vi "InjA-FPGA.vi"() -> ()   [LabVIEW 2016]
uses:
  Common-Control/Aperture Readback.ctl
  Common-Control/Glassman Readback.ctl
  Common-Control/Glassman Control.ctl
  <vilib>/LabVIEW Targets/FPGA/cRIO/shared/nicrio_ModuleControls/nicrio_cRIO-9871_BaudRateEnum.ctl
  <vilib>/LabVIEW Targets/FPGA/cRIO/shared/nicrio_ModuleControls/nicrio_cRIO-9871_DataBitsEnum.ctl
  <vilib>/LabVIEW Targets/FPGA/cRIO/shared/nicrio_ModuleControls/nicrio_cRIO-9871_ParityEnum.ctl
  <vilib>/LabVIEW Targets/FPGA/cRIO/shared/nicrio_ModuleControls/nicrio_cRIO-9871_StopBitsEnum.ctl
  <vilib>/Platform/TimedLoop/XDataNode/timing_clust.ctl
  <vilib>/Platform/TimedLoop/XDataNode/nitl_modes.ctl
  <vilib>/Platform/TimedLoop/XDataNode/wakeup.ctl
  <vilib>/rvi/FXPMathLib/basic elements/FxpIntAccumulator/subVIs/nifxpmath_IntAccumulator_SimConfig.ctl
  <vilib>/rvi/Emulation/niFpgaGetClockAttributes.vi
  <vilib>/rvi/Emulation/niFpgaSctlEmulationGetInTimedLoop.vi
  <vilib>/rvi/Emulation/niFpgaEmulationReportErrorSimple.vi
  <vilib>/rvi/eio/common/nirviEmuTemplateMethod_errors.vi
  <vilib>/rvi/Emulation/niFpgaCriticalErrorInLSC.vi
  <vilib>/rvi/Analysis/common/codeGenErrors/XNode/niFpgaXNodeCodeGenErrorHandle.vi
  <vilib>/rvi/FXPMathLib/basic elements/FxpIntAccumulator/simVIs/DllFxpIntAccumulator_sub.vi
  <vilib>/rvi/eio/common/nirviEmuTemplatePropertySet_errors.vi
  <vilib>/eio/EIONode/EIONode.xnode
  <vilib>/rvi/Analysis/measure/dc-rms/XNode/niFpgaDC-RMS.xnode
  <vilib>/Platform/TimedLoop/XDataNode/XDataNode.xnode
  <vilib>/rvi/FXPMathLib/basic elements/FxpIntAccumulator/XNode/nifxpmath_IntAccumulator.xnode
  <vilib>/rvi/FXPMathLib/FxpMul/XNode/nifxpmath_Multiplier.xnode
  <vilib>/eio/EIOPropertyNode/EIOPropertyNode.xnode
  <vilib>/Platform/TimedLoop/XDataNode/XDNodeRunTimeDep.lvlib
  <vilib>/rvi/FXPMathLib/sim/FxpSim.dll
  <vilib>/rvi/eio/common/nirviEmuTemplatePropertyGet_errors.vi
  <vilib>/rvi/eio/common/nirviEmuTemplatePropertyGet_noerrors.vi
  <vilib>/rvi/eio/common/nirviEmuTemplatePropertySet_noerrors.vi
panel:
  out "Turbo Rotation Status":bool
  out "Turbo Error Status":bool
  out "Turbo Rotation Speed":fxp<+/-,26,5>
  out "Turbo monitor loop error":errorcluster
  out "HV control loop error":errorcluster
  in  "Einzel 2 V set":T1
  in  "Y Steerer V set":T1
  in  "X Steerer V set":T1
  in  "Einzel 1 V set":T1
  out "HV readback loop error":errorcluster
  out "Y Steerer Monitor":T2
  out "X Steerer Monitor":T2
  out "Einzel 2 Monitor":T2
  out "Einzel 1 Monitor":T2
  out "Pre-Acc Aperture Position":T3
  in  "RT error":bool
  out "Vac readback loop error":errorcluster
  out "Ion gauge 1":u8[](array[numeric])
  out "Convectron 1":u8[](array[numeric])
  out "Ion gauge 2":u8[](array[numeric])
  out "Convectron 2":u8[](array[numeric])
  out "Vacuum Gauge interlock":bool
  out "Vac Interlock loop error":errorcluster
  out "Actuator Sensor loop error":errorcluster
  in  "Pre-Acc Aperture Actuator":bool
  in  "BPM 2x10":bool
  in  "BPM 2":bool
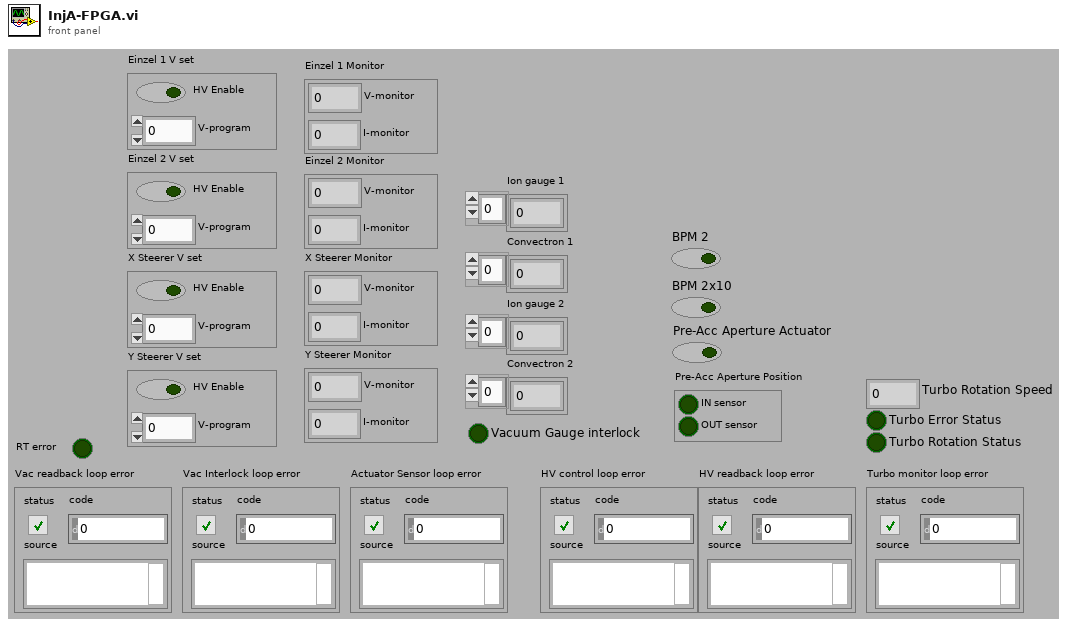
[diagram p1: front panel]
types:
  T1 = typedef "Glassman Control.ctl" = cluster{"V-program":fxp<+/-,16,5>, "HV Enable":bool}
  T2 = typedef "Glassman Readback.ctl" = cluster{"I-monitor":fxp<+/-,16,5>, "V-monitor":fxp<+/-,16,5>}
  T3 = typedef "Aperture Readback.ctl" = cluster{"IN sensor":bool, "OUT sensor":bool}
  T4 = typedef "nicrio_cRIO-9871_StopBitsEnum.ctl" = enum8{"1", "1.5", "2"}
  T5 = typedef "nicrio_cRIO-9871_ParityEnum.ctl" = enum8{"None", "Odd", "Even", "Mark", "Space"}
  T6 = typedef "nicrio_cRIO-9871_DataBitsEnum.ctl" = enum8{"5", "6", "7", "8"}
  T7 = typedef "nicrio_cRIO-9871_BaudRateEnum.ctl" = enum16{"75 bps", "110 bps", "134 bps", "150 bps", "300 bps", "600 bps", "1200 bps", "1800 bps", "2400 bps", "4800 bps", "7200 bps", "9600 bps", "14.4 kbps", "19.2 kbps", "28.8 kbps", "38.4 kbps", "57.6 kbps", "115.2 kbps", "230.4 kbps", "460.8 kbps", "921.6 kbps"}
  T8 = typedef "XDNodeRunTimeDep.lvlib/timing_clust.ctl" = cluster{"Expected End [f-1]":u64, "Actual End [f-1]":u64, "Finished Late? [f-1]":bool, "Expected End [i-1]":u64, "Actual End [i-1]":u64, "Finished Late? [i-1]":bool, "Expected Start [i]":u64, "Actual Start [i]":u64, "Expected Start [f]":u64, "Actual Start [f]":u64, "Source Name":string, "Structure Name":string, "Period":i64, "Deadline":i64, "Offset":i64, "Start":i64, "Priority":i32, "Timeout":i32, "Mode":T9, "Wakeup Reason":T10, "Error":errorcluster, "Source Type":string, "Secondary Source Type":string, "Global End Time":u64, "Global Start Time":u64, "Frame Duration":u64, "Iteration Duration":u64, "Assigned CPU":i32, "I/O Scan Engine Mode":u32}
  T9 = typedef "XDNodeRunTimeDep.lvlib/nitl_modes.ctl" = enum32{"No Change", "Process missed periods, maintain original phase", "Discard missed periods, maintain original phase", "Process missed periods, ignore original phase", "Discard missed periods, ignore original phase"}
  T10 = typedef "XDNodeRunTimeDep.lvlib/wakeup.ctl" = enum32{"Normal", "Aborted", "Asynchronous wakeup", "Timing source error", "Timed loop error", "Timeout"}
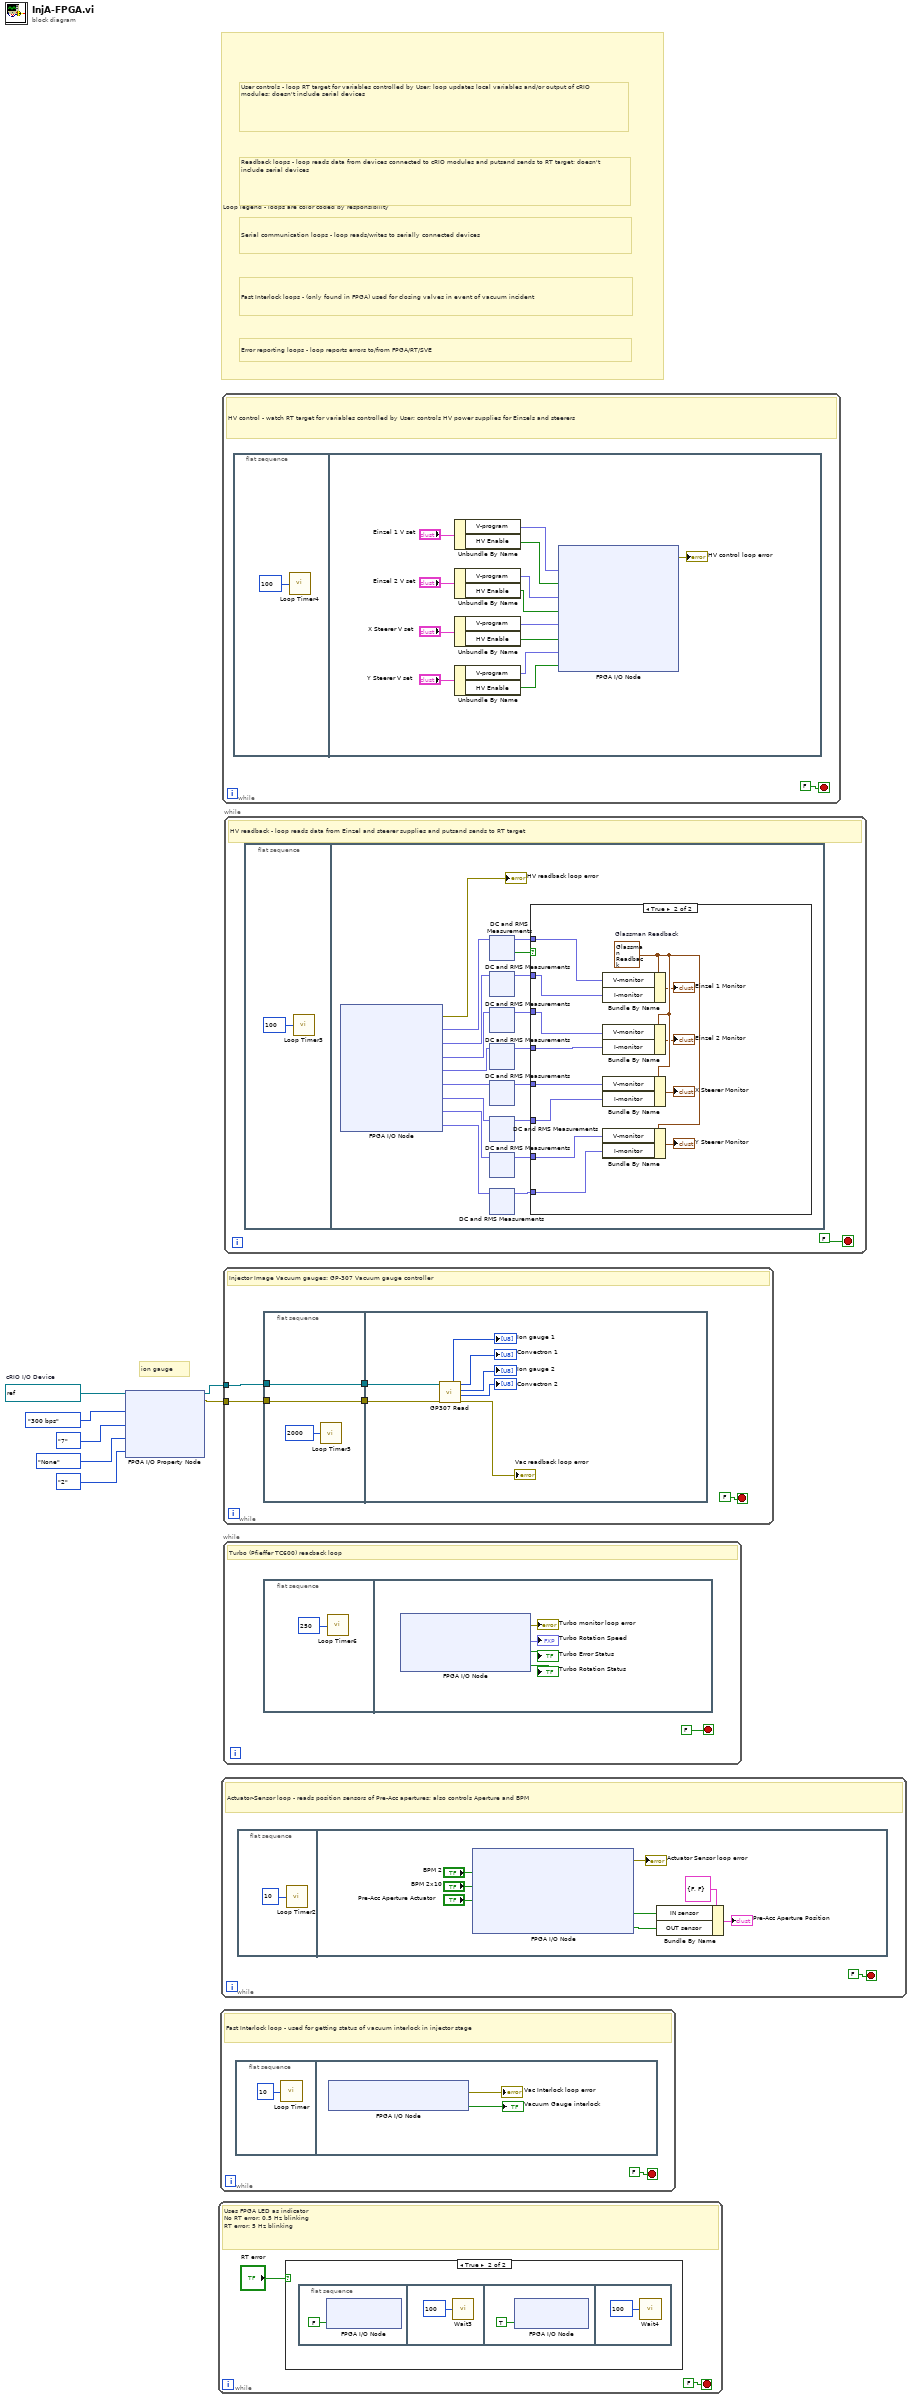
[diagram p0: block diagram]
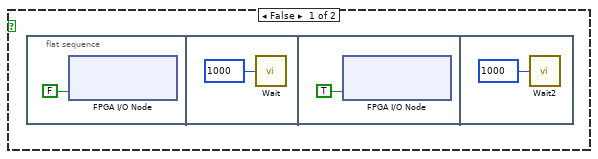
[diagram p2: hidden frame]
diagram:
  w7 = refnum<k21> "Mod8\\Port1"  # cRIO I/O Device
  # "Fast Interlock loops - (only found in FPGA) used for closing valves in event of vacuum incident"
  # "Error reporting loops - loop reports errors to/from FPGA/RT/SVE"
  # "Serial communication loops - loop reads/writes to serially connected devices"
  # "Readback loops - loop reads data from devices connected to cRIO modules and putsand sends to RT target; doesn't include serial devices"
  # "User controls - loop RT target for variables controlled by User; loop updates local variables and/or output of cRIO modules; doesn't include serial devices"
  # "Loop legend - loops are color coded by responsibility"
  # "ion gauge"
  n1 = xnode "FPGA I/O Property Node"("FPGA I/O In"=w7, "Baud Rate"=nicrio_cRIO-9871_BaudRateEnum."300 bps", "Data Bits"=nicrio_cRIO-9871_DataBitsEnum."7", "Parity"=nicrio_cRIO-9871_ParityEnum."None", "Stop Bits"=nicrio_cRIO-9871_StopBitsEnum."2") -> ("error out"=w2:errorcluster, "FPGA I/O Out"=w1:refnum<k21>)  [unwired: 1 in]
  n2 = while {
    stop <- FALSE stop-if-true
    # "Uses FPGA LED as indicator\nNo RT error: 0.5 Hz blinking\nRT error: 5 Hz blinking"
    n3 = case shown="True" "RT error" {
      frame False {
        n4 = flat-sequence {
          frame #0 {
            n5 = xnode "FPGA I/O Node"("FPGA LED"=FALSE) -> ()  [unwired: 1 in, 1 out]
          }
          frame #1 {
            n6 = call "Wait"("Count(mSec)"=u16 1000) -> ()  [unwired: 1 out]
          }
          frame #2 {
            n7 = xnode "FPGA I/O Node"("FPGA LED"=TRUE) -> ()  [unwired: 1 in, 1 out]
          }
          frame #3 {
            n8 = call "Wait2"("Count(mSec)"=u16 1000) -> ()  [unwired: 1 out]
          }
        }
      }
      frame True {
        n9 = flat-sequence {
          frame #0 {
            n10 = xnode "FPGA I/O Node"("FPGA LED"=FALSE) -> ()  [unwired: 1 in, 1 out]
          }
          frame #1 {
            n11 = call "Wait3"("Count(mSec)"=u16 100) -> ()  [unwired: 1 out]
          }
          frame #2 {
            n12 = xnode "FPGA I/O Node"("FPGA LED"=TRUE) -> ()  [unwired: 1 in, 1 out]
          }
          frame #3 {
            n13 = call "Wait4"("Count(mSec)"=u16 100) -> ()  [unwired: 1 out]
          }
        }
      }
    }
  }
  n14 = while {
    stop <- FALSE stop-if-true
    # "Fast Interlock loop - used for getting status of vacuum interlock in injector stage"
    n15 = flat-sequence {
      frame #0 {
        n16 = call "Loop Timer"("Count(uSec)"=u32 10 ("Count(Ticks)")) -> ()  [unwired: 1 out]
      }
      frame #1 {
        n17 = xnode "FPGA I/O Node"() -> ("error out"=→"Vac Interlock loop error":errorcluster, "Vacuum Gauge interlock"=→"Vacuum Gauge interlock":bool)  [unwired: 2 in, 1 out]
      }
    }
  }
  n18 = while {
    stop <- FALSE stop-if-true
    # "Actuator-Sensor loop - reads position sensors of Pre-Acc apertures; also controls Aperture and BPM"
    n19 = flat-sequence {
      frame #0 {
        n20 = call "Loop Timer2"("Count(uSec)"=u32 10 ("Count(Ticks)")) -> ()  [unwired: 1 out]
      }
      frame #1 {
        n21 = xnode "FPGA I/O Node"("BPM 2"="BPM 2", "BPM 2x10"="BPM 2x10", "Pre-Acc Aperture Actuator"="Pre-Acc Aperture Actuator") -> ("error out"=→"Actuator Sensor loop error":errorcluster, "Pre-Acc Aperture IN sensor"=w25:bool, "Pre-Acc Aperture OUT sensor"=w24:bool)  [unwired: 6 in, 5 out]
        n22 = Bundle By Name(cluster=T3 {"IN sensor"=FALSE, "OUT sensor"=FALSE} ("Aperture"), "IN sensor"=w25, "OUT sensor"=w24) -> (→"Pre-Acc Aperture Position":T3)
      }
    }
  }
  n23 = while {
    stop <- FALSE stop-if-true
    # "HV control - watch RT target for variables controlled by User; controls HV power supplies for Einzels and steerers"
    n24 = flat-sequence {
      frame #0 {
        n25 = call "Loop Timer4"("Count(mSec)"=u32 100 ("Count(Ticks)")) -> ()  [unwired: 1 out]
      }
      frame #1 {
        n26 = Unbundle By Name("Einzel 1 V set") -> ("V-program"=w35:fxp<+/-,16,5>, "HV Enable"=w36:bool)
        n27 = Unbundle By Name("Einzel 2 V set") -> ("V-program"=w37:fxp<+/-,16,5>, "HV Enable"=w38:bool)
        n28 = Unbundle By Name("X Steerer V set") -> ("V-program"=w39:fxp<+/-,16,5>, "HV Enable"=w40:bool)
        n29 = Unbundle By Name("Y Steerer V set") -> ("V-program"=w42:fxp<+/-,16,5>, "HV Enable"=w41:bool)
        n30 = xnode "FPGA I/O Node"("Einzel 1 V set"=w35, "Einzel 1 HV enable"=w36, "Einxel 2 V set"=w37, "Einzel 2 HV enable"=w38, "X steerer V set"=w39, "X steerer HV enable"=w40, "Y steerer V set"=w42, "Y steerer HV enable"=w41) -> ("error out"=→"HV control loop error":errorcluster)  [unwired: 9 in, 8 out]
      }
    }
  }
  n31 = while {
    tunnel: w2 -> [w50]
    tunnel: w1 -> [w49]
    stop <- FALSE stop-if-true
    # "Injector Image Vacuum gauges: GP-307 Vacuum gauge controller"
    n32 = flat-sequence {
      tunnel: w49 -> [w53]
      tunnel: w50 -> [w54]
      tunnel: [w54] -> w48
      tunnel: [w53] -> w47
      tunnel: w48 -> [w56]
      tunnel: w47 -> [w55]
      frame #0 {
        n33 = call "Loop Timer5"("Count(mSec)"=u32 2000 ("Count(Ticks)")) -> ()  [unwired: 1 out]
      }
      frame #1 {
        n34 = call "GP307 Read.vi"("error in"=w56, "cRIO I/O Device"=w55) -> ("error out"=→"Vac readback loop error":errorcluster, "Convectron 2"=→"Convectron 2":u8[], "Ion gauge 2"=→"Ion gauge 2":u8[], "Convectron 1"=→"Convectron 1":u8[], "Ion gauge 1"=→"Ion gauge 1":u8[])  [unwired: 5 in]
      }
    }
  }
  n35 = while {
    stop <- FALSE stop-if-true
    # "Turbo (Pfieffer TC600) reacback loop"
    n36 = flat-sequence {
      frame #0 {
        n37 = call "Loop Timer6"("Count(mSec)"=u32 250 ("Count(Ticks)")) -> ()  [unwired: 1 out]
      }
      frame #1 {
        n38 = xnode "FPGA I/O Node"() -> ("error out"=→"Turbo monitor loop error":errorcluster, "Turbo Rotation Speed"=→"Turbo Rotation Speed":fxp<+/-,26,5>, "Turbo Error Status"=→"Turbo Error Status":bool, "Turbo Rotation Status"=→"Turbo Rotation Status":bool)  [unwired: 4 in, 3 out]
      }
    }
  }
  n39 = while {
    stop <- FALSE stop-if-true
    # "HV readback - loop reads data from Einzel and steerer supplies and putsand sends to RT target"
    n40 = flat-sequence {
      frame #0 {
        n41 = call "Loop Timer3"("Count(mSec)"=u32 100 ("Count(Ticks)")) -> ()  [unwired: 1 out]
      }
      frame #1 {
        n42 = xnode "FPGA I/O Node"() -> ("error out"=→"HV readback loop error":errorcluster, "Einzel 1 V read"=w87:fxp<+/-,26,5>, "Einzel 1 I read"=w84:fxp<+/-,26,5>, "Einzel 2 V read"=w83:fxp<+/-,26,5>, "Einzel 2 I read"=w82:fxp<+/-,26,5>, "X steerer V read"=w81:fxp<+/-,26,5>, "X steerer I read"=w76:fxp<+/-,26,5>, "Y steerer V read"=w74:fxp<+/-,26,5>, "Y steerer I read"=w72:fxp<+/-,26,5>)  [unwired: 9 in, 8 out]
        n43 = xnode "DC and RMS Measurements"("input data"=w87) -> ("DC"=w85:fxp<+/-,26,5>, "output valid"=w86:bool)  [unwired: 1 in]
        n44 = xnode "DC and RMS Measurements"("input data"=w84) -> ("DC"=w80:fxp<+/-,26,5>)  [unwired: 1 in, 1 out]
        n45 = xnode "DC and RMS Measurements"("input data"=w83) -> ("DC"=w79:fxp<+/-,26,5>)  [unwired: 1 in, 1 out]
        n46 = xnode "DC and RMS Measurements"("input data"=w82) -> ("DC"=w78:fxp<+/-,26,5>)  [unwired: 1 in, 1 out]
        n47 = xnode "DC and RMS Measurements"("input data"=w81) -> ("DC"=w77:fxp<+/-,26,5>)  [unwired: 1 in, 1 out]
        n48 = xnode "DC and RMS Measurements"("input data"=w76) -> ("DC"=w75:fxp<+/-,26,5>)  [unwired: 1 in, 1 out]
        n49 = xnode "DC and RMS Measurements"("input data"=w74) -> ("DC"=w73:fxp<+/-,26,5>)  [unwired: 1 in, 1 out]
        n50 = xnode "DC and RMS Measurements"("input data"=w72) -> ("DC"=w71:fxp<+/-,26,5>)  [unwired: 1 in, 1 out]
        n51 = case shown="True" w86 {
          tunnel: w85 -> [_ w735]
          tunnel: w80 -> [_ w734]
          tunnel: w79 -> [_ w733]
          tunnel: w78 -> [_ w732]
          tunnel: w77 -> [_ w731]
          tunnel: w75 -> [_ w730]
          tunnel: w73 -> [_ w729]
          tunnel: w71 -> [_ w728]
          frame False {
          }
          frame True {
            w740 = T2 {"I-monitor"=0.0, "V-monitor"=0.0}  # Glassman Readback
            n52 = Bundle By Name(cluster=w740, "V-monitor"=w735, "I-monitor"=w734) -> (→"Einzel 1 Monitor":T2)
            n53 = Bundle By Name(cluster=w740, "V-monitor"=w733, "I-monitor"=w732) -> (→"Einzel 2 Monitor":T2)
            n54 = Bundle By Name(cluster=w740, "V-monitor"=w731, "I-monitor"=w730) -> (→"X Steerer Monitor":T2)
            n55 = Bundle By Name(cluster=w740, "V-monitor"=w729, "I-monitor"=w728) -> (→"Y Steerer Monitor":T2)
          }
        }
      }
    }
  }
